vi "Experiment header-Get parameter names-retd.vi"(8 "error in (no error)":errorcluster, 11 "Header file type":T1) -> (0 "error out":errorcluster, 3 "Parameter names":string[](array[string]))   [LabVIEW 2017]
uses:
  Typedefs/Header file type enum.ctl
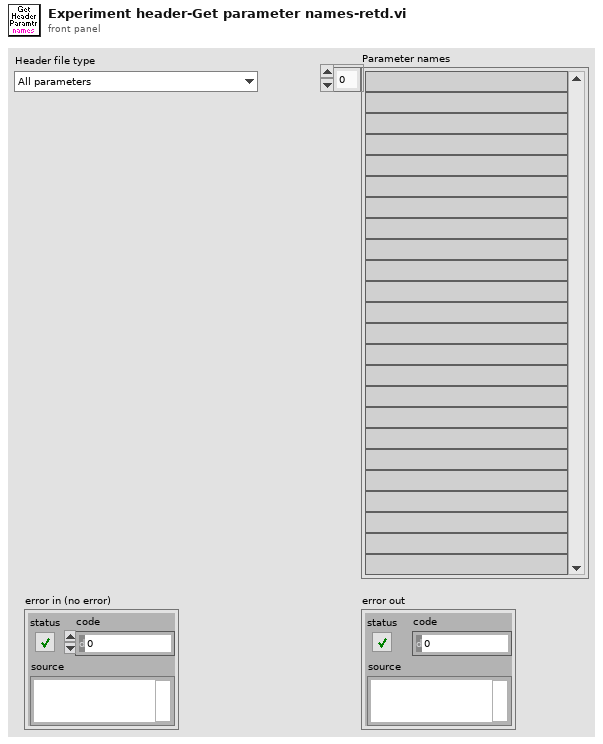
[diagram p1: front panel]
types:
  T1 = typedef "Header file type enum.ctl" = enum16{"All parameters", "Login", "Global Parameters", "Imaging Modes", "Time Series", "Motor Zstack", "AOL Zstack", "Functional Imaging", "Movement Correction", "Calibration Setup", "Statistics", "Biology Information"}
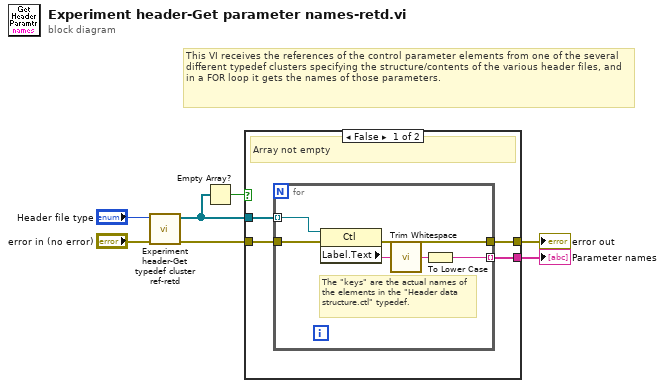
[diagram p0: block diagram]
diagram:
  # "This VI receives the references of the control parameter elements from one of the several different typedef clusters specifying the structure/contents of the various header files, and in a FOR loop it gets the names of those parameters."
  n1 = call "Experiment header-Get typedef cluster ref-retd.vi"("error in (no error)"="error in (no error)", "Header file type"="Header file type") -> ("error out"=w2:errorcluster, "Header prameter control refs[]"=w4:refnum<vi>[])  [unwired: 8 in]
  n2 = Empty Array?(array=w4) -> (empty?=w5:bool)
  n3 = case shown="False" w5 {
    tunnel: [w11 _] -> w7
    tunnel: [w10 w18] -> w6
    tunnel: w2 -> [w9 w18]
    tunnel: w4 -> [w8 _]
    frame False {
      # "Array not empty"
      n4 = for {
        tunnel: [w15] -> w11 mode=indexing
        tunnel: w9 -> [w14]
        tunnel: [w13] -> w10
        tunnel: w8 -> [w12] mode=indexing
        # "The \"keys\" are the actual names of the elements in the \"Header data structure.ctl\" typedef."
        n5 = property on="Property Node" class="Ctl"(reference=w12, error in=w14) -> (error out=w13:errorcluster, "Label.Text"=w17:string)  [unwired: 1 out]
        n6 = call <vilib>:"Trim Whitespace.vi"("string"=w17) -> ("trimmed string"=w16:string)  [unwired: 1 in]
        n7 = To Lower Case(string=w16) -> (all lower case string=w15:string)
      }
    }
    frame True {
      # "Empty array (fail-safe case)"
    }
  }
  "Parameter names" <- w7
  "error out" <- w6
